vi "ImpulseGenerator.vi"() -> ()   [LabVIEW 2014]
panel:
  in  "milliseconds to wait":u32
  in  "stop":bool
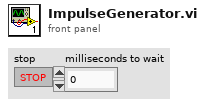
[diagram p1: front panel]
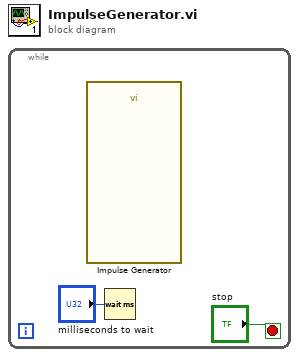
[diagram p0: block diagram]
diagram:
  n1 = while {
    stop <- "stop" stop-if-true
    n2 = call "Impulse Generator"() -> ()  [unwired: 18 in, 2 out]
    n3 = Wait (ms)(milliseconds to wait="milliseconds to wait") -> ()  [unwired: 1 out]
  }
